vi "Untitled 19 (SubVI).vi"(11 "Array in":dbl[](array[numeric])) -> (3 "Array":dbl[](array[numeric]))   [LabVIEW 2017]
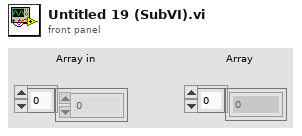
[diagram p1: front panel]
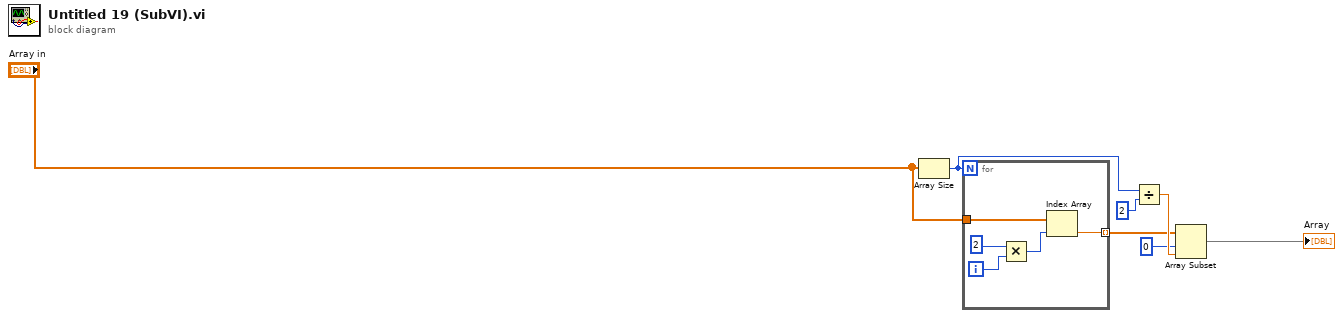
[diagram p0: block diagram]
diagram:
  n1 = Array Size(array="Array in") -> (size(s)=w3:i32)
  n2 = for {
    N: w3 -> [_]
    tunnel: "Array in" -> [w12]
    tunnel: [w9] -> w1 mode=indexing
    i -> [w10]
    n3 = Multiply(x=2, y=w10) -> (x*y=w8:i32)
    n4 = Index Array(array=w12, index=w8) -> (element=w9:dbl)
  }
  n5 = Divide(x=w3, y=2) -> (x/y=w5:dbl)
  n6 = Array Subset(array=w1, index=0, length=w5) -> (→"Array":dbl[])
